vi "TestConvert.vi"() -> ()   [LabVIEW 2020, in "Conditum-Tools.lvlib"]
uses:
  Conditum-Tools.lvlib
  Conditum-Clone/Entity ID.ctl
  <vilib>/IlluminatedG/IG Conditum Base/Conditum/Entity/Entity.lvclass
  Conditum-Clone/Entity/Entity.lvclass
  <vilib>/IlluminatedG/IG Conditum Base/Conditum/Entity ID.ctl
  <vilib>/IlluminatedG/IG Conditum Base/Conditum/Entity/Entity.lvclass/Entity.ctl
  <vilib>/IlluminatedG/IG Conditum Base/Conditum/Columns/ID/ID.lvclass/ID.ctl
  Conditum-Clone/Entity/Entity.lvclass/Entity.ctl
  Conditum-Clone/Columns/ID/ID.lvclass/ID.ctl
  a0f72350-8488-49dc-adba-a4f2f2410bf0.vi
  <vilib>/IlluminatedG/IG Conditum Base/Conditum/Columns/ID/Set.vi
  Conditum-Clone/Columns/ID/Get.vi
  <vilib>/Utility/LVClass/Get LV Class Name.vi
  <vilib>/Utility/error.llb/Error Cluster From Error Code.vi
  <vilib>/IlluminatedG/IG Conditum Base/Conditum/Conditum.lvlib
  Conditum-Clone/Conditu2.lvlib
panel:
  out "ID":T1
  out "error out":errorcluster
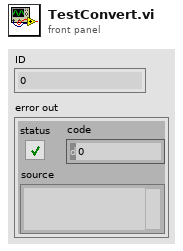
[diagram p1: front panel]
types:
  T1 = typedef "Conditu2.lvlib/Entity ID.ctl" = i64
  T2 = typedef "Conditum.lvlib/Entity ID.ctl" = i64
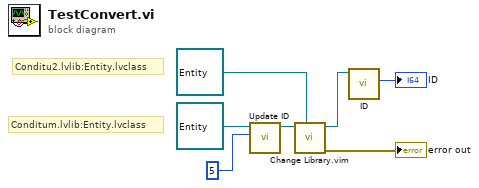
[diagram p0: block diagram]
diagram:
  # "Conditum.lvlib:Entity.lvclass"
  # "Conditu2.lvlib:Entity.lvclass"
  n1 = call <vilib>:"Update ID.vi"("Entity ID"=T2 5, "Entity in"=refnum<class "Entity.lvclass"> refnum ("Conditum:Entity")) -> ("Entity out"=w5:refnum<class "Entity.lvclass">)  [unwired: 9 in]
  n2 = call "Change Library.vim"("To Type"=refnum<class "Entity.lvclass"> refnum ("Conditum:Entity"), "From Value"=w5) -> ("error out"=→"error out":errorcluster, "To Value"=w3:refnum<class "Entity.lvclass">)  [unwired: 7 in, 1 out]
  n3 = call "ID.vi"("Entity in"=w3) -> ("ID"=→"ID":T1)  [unwired: 9 in, 1 out]
